vi "Receive Messages.vi"(8 "error in":errorcluster, 10 "Sender":string, 11 "gRPC XNET Read Raw CAN Frame Strategy in":refnum<class "gRPC XNET Read Raw CAN Frame Strategy.lvclass">) -> (0 "error out":errorcluster, 2 "Messages":refnum<class "IMessage.lvclass">[](array[class]), 3 "gRPC XNET Read Raw CAN Frame Strategy out":refnum<class "gRPC XNET Read Raw CAN Frame Strategy.lvclass">)   [LabVIEW 2024, in "gRPC XNET Read Raw CAN Frame Strategy.lvclass"]
uses:
  gRPC XNET Read Raw CAN Frame Strategy.lvclass
  Source/Interfaces/IMessage/IMessage.lvclass
  grpc-xnet/grpc-xnet_client/RPC Messages/nixnet_grpc_ReadFrameRequest_protocol_enum/nixnet_grpc_ReadFrameRequest_protocol_enum.lvclass
  grpc-xnet/grpc-xnet_client/RPC Messages/nixnet_grpc_ReadFrameRequest_timeout_enum/nixnet_grpc_ReadFrameRequest_timeout_enum.lvclass
  Source/Messages/CAN Message/CAN Message.lvclass
  D:/git/HAL/Source/Interfaces/IMessage/IMessage.lvclass
  grpc-xnet/grpc-xnet_client/RPC Messages/nixnet_grpc_ReadFrameRequest_timeout_enum/nixnet_grpc_ReadFrameRequest_timeout_enum.lvclass/nixnet_grpc_ReadFrameRequest_timeout_enum.ctl
  grpc-xnet/grpc-xnet_client/RPC Messages/nixnet_grpc_ReadFrameRequest_protocol_enum/nixnet_grpc_ReadFrameRequest_protocol_enum.lvclass/nixnet_grpc_ReadFrameRequest_protocol_enum.ctl
  gRPC XNET Read Raw CAN Frame Strategy.lvclass/gRPC XNET Read Raw CAN Frame Strategy.ctl
  grpc-xnet/grpc-xnet_client/RPC Messages/nixnet_grpc_FrameBufferResponse_frame/nixnet_grpc_FrameBufferResponse_frame.lvclass/nixnet_grpc_FrameBufferResponse_frame.ctl
  grpc-xnet/grpc-xnet_client/RPC Messages/nidevice_grpc_Session.ctl
  grpc-xnet/grpc-xnet_client/grpc-xnet_client.lvlib
  grpc-xnet/grpc-xnet_client/RPC Messages/nixnet_grpc_ReadFrameRequest.ctl
  grpc-xnet/grpc-xnet_client/RPC Messages/nixnet_grpc_Protocol.ctl
  grpc-xnet/grpc-xnet_client/RPC Messages/nixnet_grpc_TimeOut.ctl
  grpc-xnet/grpc-xnet_client/RPC Messages/nixnet_grpc_FrameBufferResponse_frame/nixnet_grpc_FrameBufferResponse_frame.lvclass
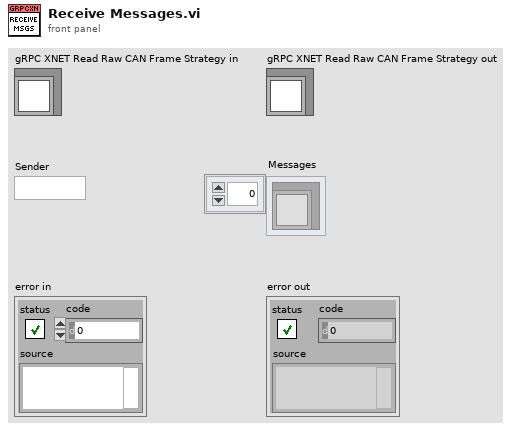
[diagram p1: front panel]
types:
  T1 = typedef "grpc-xnet_client.lvlib/nixnet_grpc_TimeOut.ctl" = enum32{"TIME_OUT_NONE", "TIME_OUT_INFINITE"}
  T2 = typedef "grpc-xnet_client.lvlib/nixnet_grpc_Protocol.ctl" = enum32{"PROTOCOL_UNSPECIFIED", "PROTOCOL_CAN", "PROTOCOL_LIN", "PROTOCOL_FLEX_RAY", "PROTOCOL_J1939", "PROTOCOL_ENET"}
  T3 = typedef "grpc-xnet_client.lvlib/nixnet_grpc_ReadFrameRequest.ctl" = cluster{"session":T4, "number_of_frames":i32, "max_payload_per_frame":u32, "nixnet_grpc_ReadFrameRequest_protocol_enum":refnum<class "nixnet_grpc_ReadFrameRequest_protocol_enum.lvclass">, "nixnet_grpc_ReadFrameRequest_timeout_enum":refnum<class "nixnet_grpc_ReadFrameRequest_timeout_enum.lvclass">}
  T4 = typedef "grpc-xnet_client.lvlib/nidevice_grpc_Session.ctl" = cluster{"name":string}
  T5 = typedef "grpc-lvsupport-release.lvlib/grpcId.ctl" = u64
  T6 = typedef "grpc-xnet_client.lvlib/nixnet_grpc_ReadFrameResponse.ctl" = cluster{"status":i32, "buffer":T7[]}
  T7 = typedef "grpc-xnet_client.lvlib/nixnet_grpc_FrameBufferResponse.ctl" = cluster{"nixnet_grpc_FrameBufferResponse_frame":refnum<class "nixnet_grpc_FrameBufferResponse_frame.lvclass">}
  T8 = typedef "grpc-xnet_client.lvlib/nixnet_grpc_FrameResponse.ctl" = cluster{"timestamp":u64, "identifier":u32, "type":T9, "type_raw":u32, "flags":T10[], "flags_raw":u32, "info":u32, "payload":u8[]}
  T9 = typedef "grpc-xnet_client.lvlib/nixnet_grpc_FrameType.ctl" = enum32{"FRAME_TYPE_CAN_DATA", "FRAME_TYPE_CAN_REMOTE", "FRAME_TYPE_CAN_BUS_ERROR", "FRAME_TYPE_CAN20_DATA", "FRAME_TYPE_CANFD_DATA", "FRAME_TYPE_CANFDBRS_DATA", "FRAME_TYPE_FLEX_RAY_DATA", "FRAME_TYPE_FLEX_RAY_NULL", "FRAME_TYPE_FLEX_RAY_SYMBOL", "FRAME_TYPE_LIN_DATA", "FRAME_TYPE_LIN_BUS_ERROR", "FRAME_TYPE_LIN_NO_RESPONSE", "FRAME_TYPE_J1939_DATA", "FRAME_TYPE_SPECIAL_DELAY", "FRAME_TYPE_SPECIAL_LOG_TRIGGER", "FRAME_TYPE_SPECIAL_START_TRIGGER"}
  T10 = typedef "grpc-xnet_client.lvlib/nixnet_grpc_FrameFlags.ctl" = enum32{"FRAME_FLAGS_UNSPECIFIED", "FRAME_FLAGS_FLEX_RAY_STARTUP", "FRAME_FLAGS_FLEX_RAY_SYNC", "FRAME_FLAGS_FLEX_RAY_PREAMBLE", "FRAME_FLAGS_FLEX_RAY_CH_A", "FRAME_FLAGS_FLEX_RAY_CH_B", "FRAME_FLAGS_LIN_EVENT_SLOT", "FRAME_FLAGS_TRANSMIT_ECHO"}
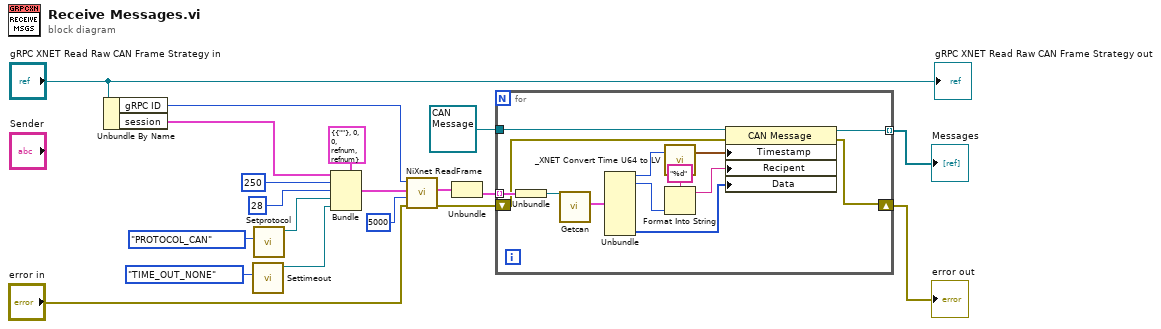
[diagram p0: block diagram]
diagram:
  n1 = Unbundle By Name("gRPC XNET Read Raw CAN Frame Strategy in") -> ("gRPC ID"=w17:T5, "session"=w18:T4)
  n2 = call "Settimeout.vi"("Set_Val"=nixnet_grpc_TimeOut."TIME_OUT_NONE") -> ("OneOfTemplate out"=w9:refnum<class "nixnet_grpc_ReadFrameRequest_timeout_enum.lvclass">)  [unwired: 9 in, 1 out]
  n3 = call "Setprotocol.vi"("Set_Val"=nixnet_grpc_Protocol."PROTOCOL_CAN") -> ("OneOfTemplate out"=w11:refnum<class "nixnet_grpc_ReadFrameRequest_protocol_enum.lvclass">)  [unwired: 9 in, 1 out]
  n4 = Bundle(cluster=T3 {"session"={"name"=""}, "number_of_frames"=0, "max_payload_per_frame"=0, "nixnet_grpc_ReadFrameRequest_protocol_enum"=refnum, "nixnet_grpc_ReadFrameRequest_timeout_enum"=refnum} ("nixnet_grpc_ReadFrameRequest"), "session"=w18, "number_of_frames"=250, "max_payload_per_frame"=u32 28, "nixnet_grpc_ReadFrameRequest_protocol_enum"=w11, "nixnet_grpc_ReadFrameRequest_timeout_enum"=w9) -> (w15:T3)
  n5 = call "NiXnet ReadFrame.vi"("error in"="error in", "timeout (ms)"=5000, "Request Data"=w15, "gRPC ID"=w17) -> ("error out"=w3:errorcluster, "Response Data"=w7:T6)  [unwired: 5 in, 1 out]
  n6 = Unbundle(w7) -> ("buffer"=w6:T7[])  [unwired: 1 out]
  n7 = for {
    tunnel: w6 -> [w32] mode=indexing
    tunnel: refnum<class "CAN Message.lvclass"> refnum ("CAN Message.lvclass") -> [w24]
    tunnel: [w23] -> w4 mode=indexing
    shift-right: [w20] -> w2
    shift-left: w3 -> [w21]
    n8 = Unbundle(w32) -> ("nixnet_grpc_FrameBufferResponse_frame"=w31:refnum<class "nixnet_grpc_FrameBufferResponse_frame.lvclass">)
    n9 = call "Getcan.vi"("OneOfTemplate in"=w31) -> ("Get_Val"=w30:T8)  [unwired: 8 in, 2 out]
    n10 = Unbundle(w30) -> ("timestamp"=w29:u64, "identifier"=w26:u32, "payload"=w27:u8[])  [unwired: 5 out]
    n11 = call <vilib>:"_XNET Convert Time U64 to LV.vi"("Time U64"=w29) -> ("Time LV"=w28:timestamp)  [unwired: 2 in]
    n12 = Format Into String(format string="%d", w26) -> (resulting string=w25:string)  [unwired: 2 in, 1 out]
    n13 = property class="CAN Message"(reference=w24, error in=w21, "Timestamp"=w28, "Recipent"=w25, "Data"=w27) -> (reference out=w23:refnum<class "CAN Message.lvclass">, error out=w20:errorcluster)
  }
  "error out" <- w2
  "Messages" <- w4
  "gRPC XNET Read Raw CAN Frame Strategy out" <- "gRPC XNET Read Raw CAN Frame Strategy in"
